vi "AddTCPCommands&Responses_GIS Printer.vi"(8 "error in (no error)":errorcluster, 10 "Command \\ Response":string[](array[string]), 11 "GIS Printer In":refnum<class "GIS Printer.lvclass">) -> (0 "error out":errorcluster, 3 "GIS Printer Out":refnum<class "GIS Printer.lvclass">)   [LabVIEW 2022 SP3, in "GIS Printer.lvclass"]
uses:
  GIS Printer.lvclass
  GIS Printer.lvclass/GIS Printer.ctl
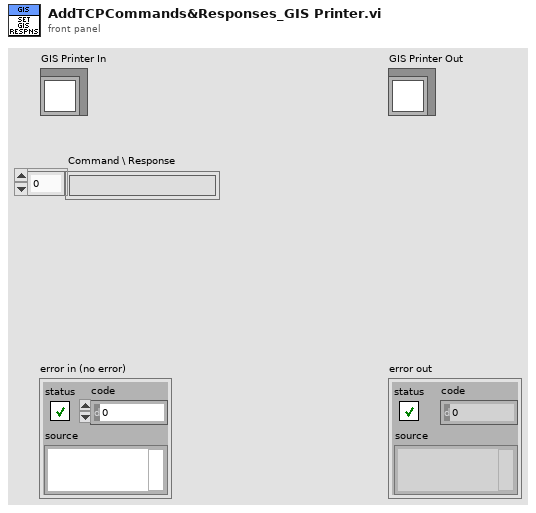
[diagram p1: front panel]
types:
  T1 = typedef "GIS Printer.lvclass/Private Data.ctl" = cluster{"UserEvents":T2, "All Dependencies":cluster{"Class References":refnum<class>[], "Class Names":string[]}, "PrinterConiguration":T3, "Status":T4, "GISHeadStatus":T5[], "HeadStatus":T6}
  T2 = typedef "GIS Printer.lvclass/UserEvents.ctl" = cluster{"API Incoming Event":refnum<user-event>, "API Executed Event":refnum<user-event>, "API Return Event":refnum<user-event>, "Status Changed Event":refnum<user-event>, "Abort":refnum<user-event>, "stop process":refnum<user-event>, "GISPollStatus":refnum<user-event>, "GISHeadStatus":refnum<user-event>, "Error Event":refnum<user-event>}
  T3 = typedef "GIS Printer.lvclass/PrinterConfiguration--Cluster.ctl" = cluster{"IPAddress":string, "Move Stage on RTP Command?":bool, "Stage Move Position":string, "PH1-Prime Path":path, "PH2-Prime Path":path, "PH3-Prime Path":path, "PH4-Prime Path":path, "PH5-Prime Path":path, "PH6-Prime Path":path, "PrintScriptsFolder":path, "PurgeScriptsFolder":path, "StageScriptsFolder":path, "PH1-HeatOn Path":path, "PH2-HeatOn Path":path, "PH3-HeatOn Path":path, "PH4-HeatOn Path":path, "PH5-HeatOn Path":path, "PH6-HeatOn Path":path, "PH1-HeatOff Path":path, "PH2-HeatOff Path":path, "PH3-HeatOff Path":path, "PH4-HeatOff Path":path, "PH5-HeatOff Path":path, "PH6-HeatOff Path":path}
  T4 = typedef "GIS Printer.lvclass/Status Cluster.ctl" = cluster{"Command Status":variant, "TCP Commands & Responses":string[][], "Printer Busy?":bool}
  T5 = typedef "GIS Status--Cluster.ctl" = cluster{"HeadEnabled":bool, "SpitEnabled":bool, "HeaterEnabled":bool, "TargetTemperature":dbl, "CurrentTemperature":dbl}
  T6 = typedef "HeadEnableStatus--cluster.ctl" = cluster{"PH1_Enable":bool, "PH2_Enable":bool, "PH3_Enable":bool, "PH4_Enable":bool, "PH5_Enable":bool, "PH6_Enable":bool}
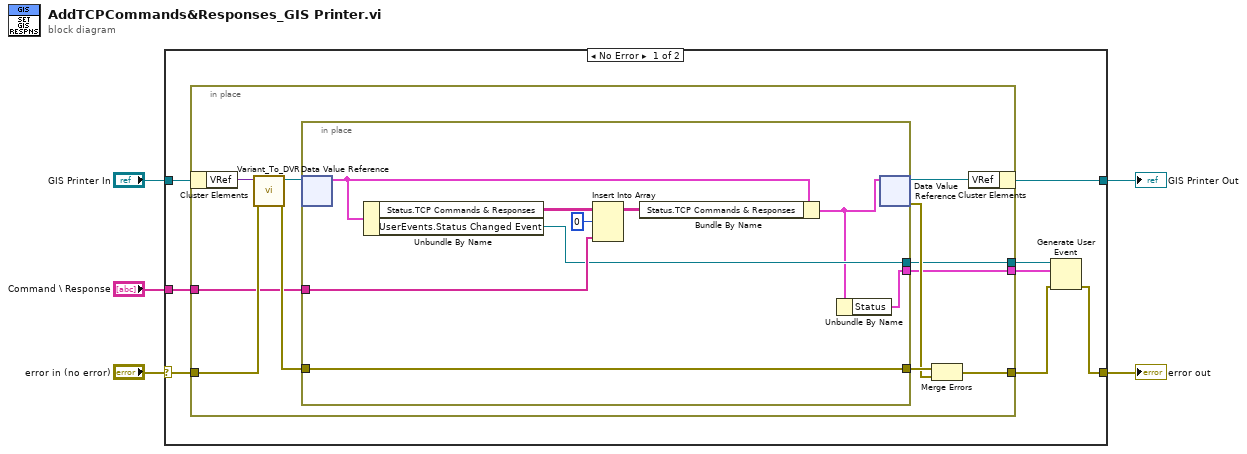
[diagram p0: block diagram]
diagram:
  n1 = case shown="No Error" "error in (no error)" {
    selector: "error in (no error)" -> [w11 w35]
    tunnel: [w7 w35] -> w4
    tunnel: [w13 w34] -> w2
    tunnel: "GIS Printer In" -> [w12 w34]
    tunnel: "Command \\ Response" -> [w10 _]
    frame No Error {
      n2 = in-place {
        in-place-border: w11 -> [w22]
        in-place-border: [w18] -> w8
        in-place-border: w10 -> [w16]
        in-place-border: [w15] -> w9
        in-place-border: [w14] -> w6
        n3 = in-place-cluster #1(w12) -> ("VRef"=w24:variant)
        n4 = call "Variant_To_DVR.vi"("error in (no error)"=w22, "Variant"=w24) -> ("error out"=w21:errorcluster, "DVR"=w23:refnum<data-value>)  [unwired: 8 in]
        n5 = in-place {
          in-place-border: w21 -> [w33]
          in-place-border: [w33] -> w20
          in-place-border: w16 -> [w29]
          in-place-border: [w28] -> w15
          in-place-border: [w25] -> w14
          n6 = in-place-dvr #2(w23) -> (w32:T1)  [unwired: 1 out]
          n7 = Unbundle By Name(w32) -> ("Status.TCP Commands & Responses"=w31:string[][], "UserEvents.Status Changed Event"=w28:refnum<user-event>)
          n8 = Insert Into Array(array=w31, index (row)=0, new element=w29) -> (w30:string[][])  [unwired: 1 in]
          n9 = Bundle By Name(cluster=w32, "Status.TCP Commands & Responses"=w30) -> (w26:T1)
          n10 = Unbundle By Name(w26) -> ("Status"=w25:T4)
          n11 = in-place-dvr #2(w26) -> (w17:refnum<data-value>, w19:errorcluster)
        }
        n12 = Merge Errors(w20, w19) -> (w18:errorcluster)
        n13 = in-place-cluster #1("VRef"=w17) -> (w13:refnum<class "GIS Printer.lvclass">)
      }
      n14 = Generate User Event(user event=w9, event data cluster=w6, error in=w8) -> (error out=w7:errorcluster)  [unwired: 1 in, 1 out]
    }
    frame Error {
    }
  }
  "error out" <- w4
  "GIS Printer Out" <- w2
